vi "Global - Keyboard Commands.vi"(7 "Mode":enum16{"Initialize", "Read", "Write"}(ring), 9 "error in (no error)":errorcluster, 10 "X, Y, Theta command (in)":dbl[](array[numeric])) -> (1 "error out":errorcluster, 2 "X, Y, Theta command (out)":dbl[](array[numeric]))   [LabVIEW 2017]
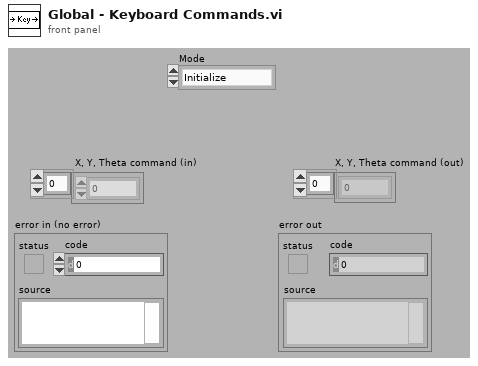
[diagram p1: front panel]
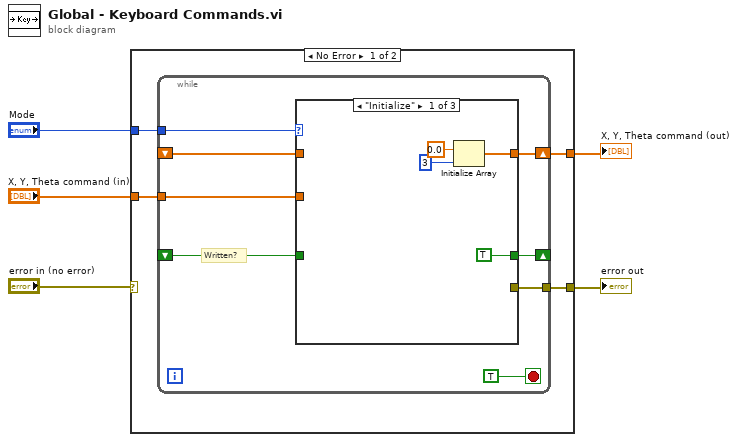
[diagram p0: block diagram]
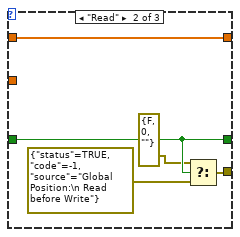
[diagram p2: hidden frame]
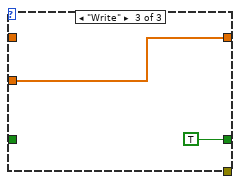
[diagram p3: hidden frame]
diagram:
  n1 = case shown="No Error" "error in (no error)" {
    selector: "error in (no error)" -> [_ w29]
    tunnel: [w6 w29] -> w4
    tunnel: "Mode" -> [w9 _]
    tunnel: "X, Y, Theta command (in)" -> [w8 _]
    tunnel: [w7 _] -> w1
    frame No Error {
      n2 = while {
        shift-right: [w14] -> w7
        shift-left: _ -> [w11]
        shift-right: [w15] -> _
        shift-left: _ -> [w12]
        tunnel: w9 -> [w16]
        tunnel: w8 -> [w13]
        tunnel: [w10] -> w6
        stop <- TRUE stop-if-true
        # "Written?"
        n3 = case shown="\"Initialize\"" w16 {
          tunnel: [TRUE w25 TRUE] -> w15
          tunnel: [w19 w26 w27] -> w14
          tunnel: w13 -> [_ _ w27]
          tunnel: w12 -> [_ w25 _]
          tunnel: w11 -> [_ w26 _]
          tunnel: [_ w22 _] -> w10
          frame "Initialize" {
            n4 = Initialize Array(0.0 ("element"), 3 ("dimension size")) -> (w19:dbl[])
          }
          frame "Read" {
            n5 = Select(t=errorcluster {"status"=FALSE, "code"=0, "source"=""}, s=w25, f=errorcluster {"status"=TRUE, "code"=-1, "source"="Global Position:\n Read before Write"} ("error IO")) -> (s? t:f=w22:errorcluster)
          }
          frame "Write" {
          }
        }
      }
    }
    frame Error {
    }
  }
  "X, Y, Theta command (out)" <- w1
  "error out" <- w4
